vi "Format Error Message.vi"(8 "error in (no error)":errorcluster, 11 "Date / Time":string) -> (2 "Error Substring":string, 3 "Error Message":string)   [LabVIEW 2012, in "OpenCLV x64.lvlib"]
uses:
  OpenCLV x64.lvlib
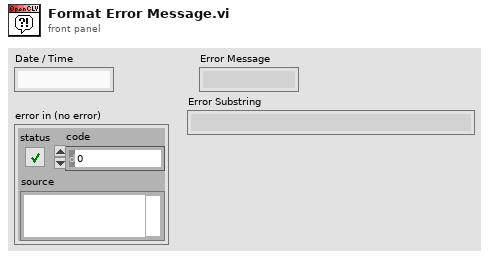
[diagram p1: front panel]
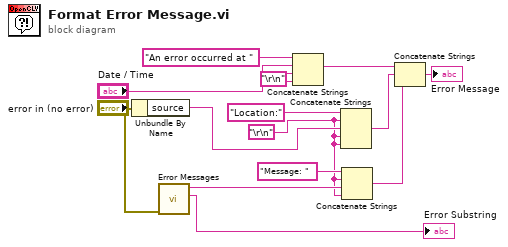
[diagram p0: block diagram]
diagram:
  w1 = "\r\n"
  w3 = "\r\n"
  n1 = Unbundle By Name("error in (no error)") -> ("source"=w7:string)
  n2 = call "Error Messages.vi"("error in (no error)"="error in (no error)") -> ("Error Substring"=→"Error Substring":string, "message"=w9:string)  [unwired: 9 in]
  n3 = Concatenate Strings("An error occurred at " ("string"), "Date / Time", w3, w3) -> (w10:string)
  n4 = Concatenate Strings("Location:" ("string"), w1, w7, w1, w1) -> (w11:string)
  n5 = Concatenate Strings("Message: " ("string"), w1, w9, w1) -> (w12:string)
  n6 = Concatenate Strings(w10, w11, w12) -> (→"Error Message":string)
